vi "Verify Waveform MD5.vi"(6 "error in":errorcluster, 9 "filename":path=path "C:/5-01-003 Active Electrode Min Max/xx Waveform 1.dat") -> (0 "error out":errorcluster, 1 "calculated MD5":string, 2 "file MD5":string, 4 "MD5 correct":bool)   [LabVIEW 2010]
doc: "This function verifies the MD5 message-digest in a waveform file."
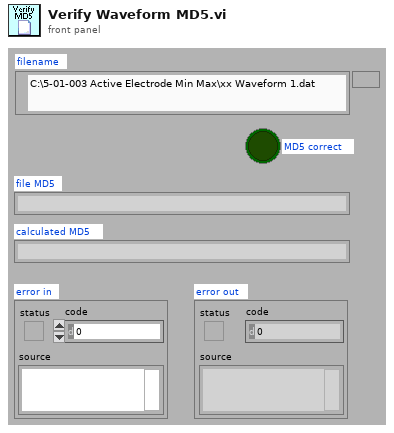
[diagram p1: front panel]
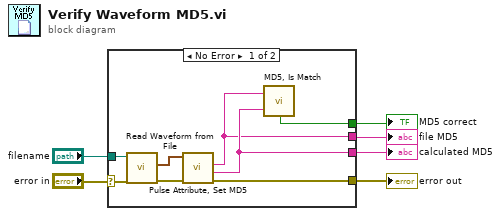
[diagram p0: block diagram]
diagram:
  n1 = case shown="No Error" "error in" {
    selector: "error in" -> [w14 w15]
    tunnel: [w10 w15] -> w5
    tunnel: "filename" -> [w13 _]
    tunnel: [w8 _] -> w4
    tunnel: [w9 _] -> w2
    tunnel: [w7 _] -> w1
    frame No Error {
      n2 = call <vilib>:"Read Waveform from File.vi"("error in (no error)"=w14, "file path (dialog if empty)"=w13) -> ("error out"=w12:errorcluster, "first waveform in record"=w11:waveform(dbl))  [unwired: 4 in, 2 out]
      n3 = call "Pulse Attribute, Set MD5.vi"("error in"=w12, "waveform"=w11) -> ("error out"=w10:errorcluster, "New MD5"=w9:string, "Old MD5"=w8:string)  [unwired: 3 in, 2 out]
      n4 = call "MD5, Is Match.vi"("MD5(b)"=w9, "MD5(a)"=w8) -> ("MD5 match"=w7:bool)  [unwired: 5 out]
    }
    frame Error {
    }
  }
  "error out" <- w5
  "calculated MD5" <- w2
  "file MD5" <- w4
  "MD5 correct" <- w1
